vi "WriteDeviceState.vi"(8 "error in (no error)":errorcluster, 10 "DeviceState (5=RUN, 6=STOP)":i16, 11 "AdsNET in":refnum<class "AdsNET.lvclass">) -> (0 "error out":errorcluster, 3 "AdsNET out":refnum<class "AdsNET.lvclass">)   [LabVIEW 2016, in "TCatAdsNet.lvlib" / "AdsNET.lvclass"]
doc: "Write Device State"
uses:
  AdsNET.lvclass
  AdsNET.lvclass/AdsNET.ctl
  C:/Users/Maurizio/Projects/twincat-lv-ads-library/TCatAdsNet Library/TwinCAT.Ads.dll
  TwinCAT.Ads.dll
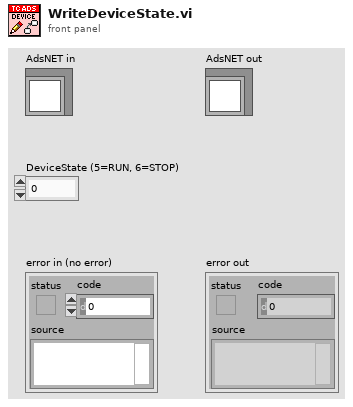
[diagram p1: front panel]
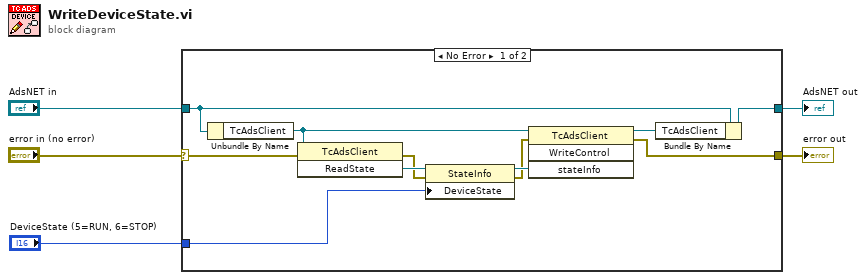
[diagram p0: block diagram]
diagram:
  n1 = case shown="No Error" "error in (no error)" {
    selector: "error in (no error)" -> [w8 w18]
    tunnel: [w11 w18] -> w4
    tunnel: [w15 w17] -> w2
    tunnel: "AdsNET in" -> [w16 w17]
    tunnel: "DeviceState (5=RUN, 6=STOP)" -> [w6 _]
    frame No Error {
      n2 = Unbundle By Name(w16) -> ("TcAdsClient"=w10:refnum<k24>)
      n3 = invoke class="TcAdsClient" method="ReadState"(reference=w10, error in=w8) -> (error out=w7:errorcluster, "ReadState"=w9:refnum<k24>)  [unwired: 1 in, 1 out]
      n4 = property class="StateInfo"(reference=w9, error in=w7, "DeviceState"=w6) -> (reference out=w13:refnum<k24>, error out=w12:errorcluster)
      n5 = invoke class="TcAdsClient" method="WriteControl"(reference=w10, error in=w12, "stateInfo"=w13) -> (reference out=w14:refnum<k24>, error out=w11:errorcluster)  [unwired: 1 in, 2 out]
      n6 = Bundle By Name(cluster=w16, "TcAdsClient"=w14) -> (w15:refnum<class "AdsNET.lvclass">)
    }
    frame Error {
    }
  }
  "error out" <- w4
  "AdsNET out" <- w2
